vi "Report Gen Section Header.vi"(8 "error in (no error)":errorcluster, 9 "Section Text":string, 10 "Section Title":string, 11 "report":T1) -> (0 "error out":errorcluster, 3 "report out":T1)   [LabVIEW 2020, in "WebServiceImporter.lvlib" / "Error Handling.lvlib"]
uses:
  <vilib>/Platform/WebService/Error Handling/Error Handling.lvlib
  <resource>/importtools/NISH Report/Generate Report Object Reference.ctl
  <resource>/importtools/NISH Report/NISH Report.lvlib
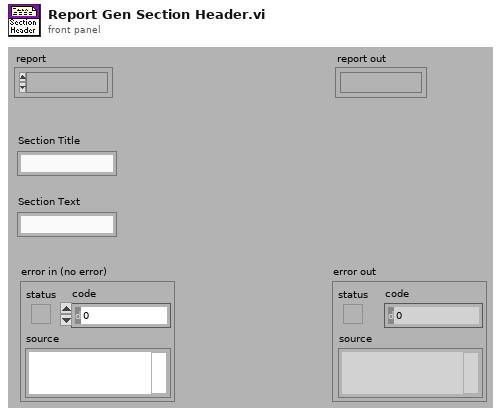
[diagram p1: front panel]
types:
  T1 = typedef "NISH Report.lvlib/Generate Report Object Reference.ctl" = refnum<k1>
  T2 = cluster{"Italic":enum16{"Italic Unchanged", "Italic On", "Italic Off"}, "Strike Through":enum16{"Strike Through Unchanged", "Strike Through On", "Strike Through Off"}, "Underline":enum16{"Underline Unchanged", "Underline On", "Underline Off"}, "Bold":enum16{"Bold Unchanged", "Bold On", "Bold Off"}}
  T3 = cluster{"Charset (-1)":i16, "Weight (-1)":i16, "Name":string, "Size":string}
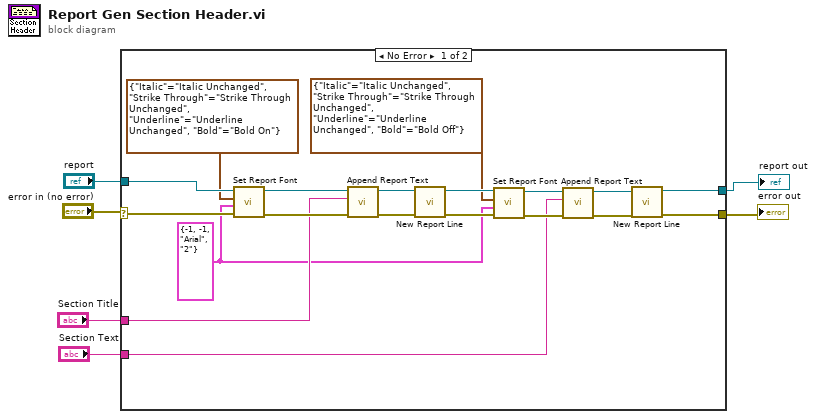
[diagram p0: block diagram]
diagram:
  n1 = case shown="No Error" "error in (no error)" {
    selector: "error in (no error)" -> [w25 w26]
    tunnel: "report" -> [w24 w27]
    tunnel: "Section Title" -> [w20 _]
    tunnel: "Section Text" -> [w11 _]
    tunnel: [w8 w26] -> w2
    tunnel: [w7 w27] -> w1
    frame No Error {
      w14 = T3 {"Charset (-1)"=-1, "Weight (-1)"=-1, "Name"="Arial", "Size"="2"} ("Font Settings")
      n2 = call <resource>:"Set Report Font.vi"("error in (no error)"=w25, "font settings"=w14, "text options"=T2 {"Italic"=enum."Italic Unchanged", "Strike Through"=enum."Strike Through Unchanged", "Underline"=enum."Underline Unchanged", "Bold"=enum."Bold On"} ("Text Options"), "report in"=w24) -> ("error out"=w22:errorcluster, "report out"=w21:T1)  [unwired: 3 in]
      n3 = call <resource>:"Append Report Text.vi"("error in (no error)"=w22, "text"=w20, "report in"=w21) -> ("error out"=w19:errorcluster, "report out"=w18:T1)  [unwired: 3 in]
      n4 = call <resource>:"New Report Line.vi"("error in (no error)"=w19, "report in"=w18) -> ("error out"=w17:errorcluster, "report out"=w16:T1)  [unwired: 4 in]
      n5 = call <resource>:"Set Report Font.vi"("error in (no error)"=w17, "font settings"=w14, "text options"=T2 {"Italic"=enum."Italic Unchanged", "Strike Through"=enum."Strike Through Unchanged", "Underline"=enum."Underline Unchanged", "Bold"=enum."Bold Off"} ("Text Options"), "report in"=w16) -> ("error out"=w13:errorcluster, "report out"=w12:T1)  [unwired: 3 in]
      n6 = call <resource>:"Append Report Text.vi"("error in (no error)"=w13, "text"=w11, "report in"=w12) -> ("error out"=w10:errorcluster, "report out"=w9:T1)  [unwired: 3 in]
      n7 = call <resource>:"New Report Line.vi"("error in (no error)"=w10, "report in"=w9) -> ("error out"=w8:errorcluster, "report out"=w7:T1)  [unwired: 4 in]
    }
    frame Error {
    }
  }
  "report out" <- w1
  "error out" <- w2
